vi "load_fp_openg.vi"(8 "error in (no error)":errorcluster, 11 "VI in":refnum<vi>) -> (0 "error out":errorcluster)   [LabVIEW 2018]
uses:
  <vilib>/Utility/config.llb/NI_LVConfig.lvlib
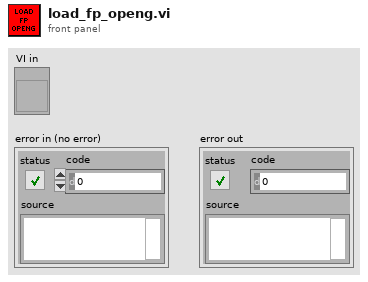
[diagram p1: front panel]
types:
  T1 = typedef "NI_LVConfig.lvlib/Config Data RefNum.ctl" = refnum<k1>
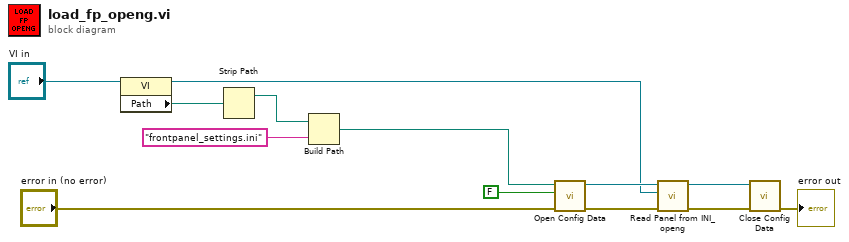
[diagram p0: block diagram]
diagram:
  n1 = property class="VI"(reference="VI in") -> (reference out=w9:refnum<vi>, "Path"=w1:path)  [unwired: 1 in, 1 out]
  n2 = Strip Path(path=w1) -> (stripped path=w3:path)  [unwired: 1 out]
  n3 = Build Path(base path=w3, name or relative path="frontpanel_settings.ini") -> (appended path=w5:path)
  n4 = call <vilib>:"Open Config Data.vi"("error in (no error)"="error in (no error)", "create file if necessary (T)"=FALSE, "configuration file path"=w5) -> ("error out"=w7:errorcluster, "refnum"=w10:T1)  [unwired: 6 in, 1 out]
  n5 = call <userlib>:"Read Panel from INI_openg.vi"("error in (no error)"=w7, "VI ref"=w9, "refnum"=w10) -> ("error out"=w8:errorcluster, "refnum out"=w11:T1)  [unwired: 7 in]
  n6 = call <vilib>:"Close Config Data.vi"("error in (no error)"=w8, "refnum"=w11) -> ("error out"=→"error out":errorcluster)  [unwired: 8 in, 1 out]
